vi "Client Test.vi"() -> ()   [LabVIEW 2013]
uses:
  SSL_Lib/SSL-Lib/SSL-Lib.lvclass
  SSL_Lib/SSL-Context/SSL-Context.lvclass
  SSL_Lib/BIO/BIO.lvclass
  SSL_Lib/SSL/SSL.lvclass
panel:
  out "*BIO":u64
  out "*SSL":u64
  out "ssl_new_ctx":string
  out "bio_new_ssl_connect":string
  out "get_ssl":string
  out "return type 2":u32
  out "error code":u32
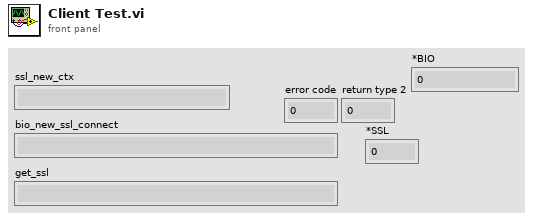
[diagram p1: front panel]
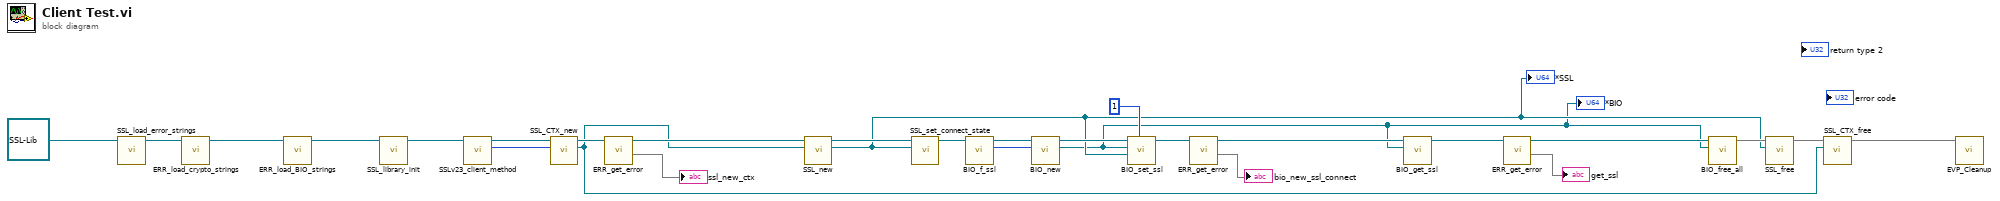
[diagram p0: block diagram]
diagram:
  n1 = call "SSL_load_error_strings.vi"("SSL-Lib in"=refnum<class "SSL-Lib.lvclass"> refnum ("SSL_Lib in")) -> ("SSL-Lib out"=w27:refnum<class "SSL-Lib.lvclass">)  [unwired: 9 in, 1 out]
  n2 = call "ERR_load_crypto_strings.vi"("SSL-Lib in"=w27) -> ("SSL-Lib out"=w13:refnum<class "SSL-Lib.lvclass">)  [unwired: 9 in, 1 out]
  n3 = call "ERR_load_BIO_strings.vi"("SSL-Lib in"=w13) -> ("SSL-Lib out"=w12:refnum<class "SSL-Lib.lvclass">)  [unwired: 9 in, 1 out]
  n4 = call "SSL_library_init.vi"("SSL-Lib in"=w12) -> ("SSL-Lib out"=w26:refnum<class "SSL-Lib.lvclass">)  [unwired: 9 in, 1 out]
  n5 = call "SSLv23_client_method.vi"("SSL-Lib in"=w26) -> ("*SSL_Method"=w25:u64, "SSL-Lib out"=w24:refnum<class "SSL-Lib.lvclass">)  [unwired: 8 in, 1 out]
  n6 = call "SSL_CTX_new.vi"("*SSL_Method"=w25, "SSL-Lib in"=w24) -> ("SSL-Context out"=w14:refnum<class "SSL-Context.lvclass">, "SSL-Lib out"=w23:refnum<class "SSL-Lib.lvclass">)  [unwired: 7 in, 1 out]
  n7 = call "ERR_get_error.vi"("SSL-Lib in"=w23) -> (1:→"ssl_new_ctx", "SSL-Lib out"=w15:refnum<class "SSL-Lib.lvclass">)  [unwired: 8 in, 1 out]
  n8 = call "SSL_new.vi"(10:w14, "SSL-Context in"=w15) -> ("SSL out"=w2:refnum<class "SSL.lvclass">, "SSL-Context out"=w11:refnum<class "SSL-Context.lvclass">)  [unwired: 7 in, 1 out]
  "*SSL" <- w2
  n9 = call "SSL_set_connect_state.vi"(10:w2, "SSL-Lib in"=w11) -> ("SSL-Lib out"=w10:refnum<class "SSL.lvclass">)  [unwired: 8 in, 1 out]
  n10 = call "BIO_f_ssl.vi"("SSL-Lib in"=w10) -> ("*BIO_Method"=w8:u64, "SSL-Lib out"=w9:refnum<class "SSL.lvclass">)  [unwired: 8 in, 1 out]
  n11 = call "BIO_new.vi"("*BIO_method"=w8, "SSL-Lib in"=w9) -> ("BIO out"=w1:refnum<class "BIO.lvclass">, "SSL-Lib out"=w7:refnum<class "SSL.lvclass">)  [unwired: 7 in, 1 out]
  "*BIO" <- w1
  n12 = call "BIO_set_ssl.vi"("close flag"=1, 9:w2, "SSL in"=w1, "BIO in"=w7) -> ("BIO out"=w5:refnum<class "BIO.lvclass">)  [unwired: 6 in, 1 out]
  n13 = call "ERR_get_error.vi"("SSL-Lib in"=w5) -> (1:→"bio_new_ssl_connect", "SSL-Lib out"=w16:refnum<class "BIO.lvclass">)  [unwired: 8 in, 1 out]
  n14 = call "BIO_get_ssl.vi"(10:w1, "BIO in"=w16) -> ("BIO out"=w20:refnum<class "BIO.lvclass">)  [unwired: 7 in, 2 out]
  n15 = call "ERR_get_error.vi"("SSL-Lib in"=w20) -> (1:→"get_ssl", "SSL-Lib out"=w19:refnum<class "BIO.lvclass">)  [unwired: 8 in, 1 out]
  n16 = call "BIO_free_all.vi"(10:w1, "BIO in"=w19) -> (3:w3)  [unwired: 8 in, 1 out]
  n17 = call "SSL_free.vi"(10:w2, "SSL in"=w3) -> (3:w4)  [unwired: 8 in, 1 out]
  n18 = call "SSL_CTX_free.vi"(10:w14, "SSL-Context in"=w4) -> (3:w22)  [unwired: 8 in, 1 out]
  n19 = call "EVP_Cleanup.vi"("SSL-Lib in"=w22) -> ()  [unwired: 9 in, 2 out]
